vi "Write Trace Controller.vi"(8 "error in (no error)":errorcluster, 9 "Trace Level":T1(ring)=enum."Informational", 10 "Trace Controller":refnum<class "Message Enqueuer.lvclass">, 11 "System Actor in":refnum<class "System Actor.lvclass">) -> (0 "error out":errorcluster, 3 "System Actor out":refnum<class "System Actor.lvclass">)   [LabVIEW 2014, in "Robot Actor Framework.lvlib" / "System Actor.lvlib" / "System Actor.lvclass"]
uses:
  System Actor.lvclass
  <vilib>/ActorFramework/Message Enqueuer/Message Enqueuer.lvclass
  System Actor.lvclass/System Actor.ctl
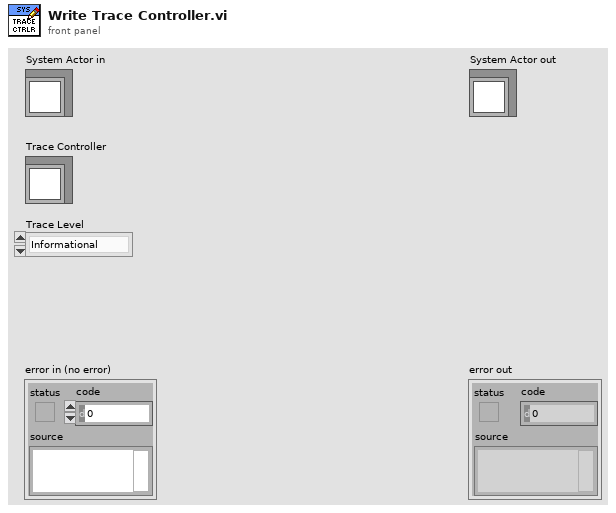
[diagram p1: front panel]
types:
  T1 = enum16{"Critical", "Error", "Warning", "Informational", "Debug"}
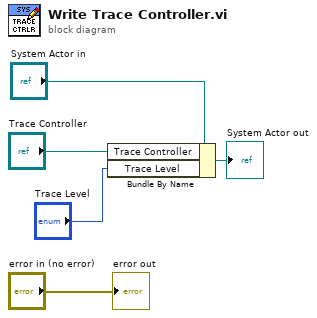
[diagram p0: block diagram]
diagram:
  n1 = Bundle By Name(cluster="System Actor in", "Trace Controller"="Trace Controller", "Trace Level"="Trace Level") -> (→"System Actor out":refnum<class "System Actor.lvclass">)
  "error out" <- "error in (no error)"
